vi "FTMS.vi"() -> ()   [LabVIEW 2011]
doc: "Enables and disables RF output of PSG1 & PSG2"
uses:
  Hardware Control/OSC/SubVIs/controls/sampling_rate.ctl
  Hardware Control/OSC/SubVIs/controls/scale.ctl
  global.vi
panel:
  out "frame averages completed:":i32 caption="averages:"
  in  "frame single cycle":bool caption="no averaging"
  in  "reset frame average":bool
  in  "Frame":i32=1 caption="Displayed Frame" min=1 step=1
  out "OSC reading":bool
  in  "meas cluster":T1
  out "waiting":bool
  in  "Pause":bool
  in  "Stop":bool
  out "current step":i32
  out "current frequency":dbl format="%6.2p"
  out "current meas cycle":i32
  out "dt":dbl format="%#_6p"
  out "reset meas cycle timer":bool
  out "first start":bool
  in  "Tab Control":T2(tab)
  in  "EXP chirp end":dbl=1000000000.0 format="%.2p"
  in  "EXP Meas Period (s)":dbl=10.0 min=1.0 format="%.2g"
  in  "Purge Freq.":dbl=2.0 caption="Purge Freq. (Hz)"
  in  "PURGE nozzle":bool
  in  "Refresh meas time":bool
  out "meas cycle time (ms)":u32
  in  "start experiment":bool
  in  "config TRIG":bool
  in  "config OSC":bool
  out "OSC resolution":ext=24999.999999999999998 caption="spectral resolution (Hz)" format="%#_6p"
  out "OSC sample points":i32=200000 caption="points / frame"
  out "TRIG BG cycle":dbl=100.0 caption="BG. cycle" min=0.0 max=999.999999999995 format="%.2p"
  out "TRIG mol delay":dbl=9.999999999999999e-05 caption="Mol. delay" min=0.0 max=999.999999999995 format="%.2p"
  out "TRIG start time":dbl[](array[numeric])=[0.0, 1.1e-06, 6.6e-06, 6.4e-06] caption="delay starts (s)" format="%.3p"
  out "TRIG burst enable":bool=TRUE caption="Burst"
  out "TRIG delay duration":dbl=4.6625e-05 caption="delay cycle (s)" format="%.2p"
  out "TRIG duration":dbl[](array[numeric])=[5.65e-06, 4.9999999999999996e-06, 4e-05, 4.9999999999999996e-06] caption="delay durations (s)" min=0.0 format="%.3p"
  out "TRIG burst period":dbl=4.9999999999999975e-05 caption="burst period (s)" format="%.2p"
  out "TRIG burst count":i32=1 caption="burst count"
  out "horizontal scale":T3=4e-06 items=["400ns/div"=4e-07, "1µs/div"=1e-06, "2µs/div"=2e-06, "4µs/div"=4e-06, "10µs/div"=1e-05, "20µs/div"=2e-05]
  out "sample rate":T4=5000000000.0 items=["20 GHz (50ps/sample)", "10 GHz (100ps/sample)", "5.0 GHz (200ps/sample)", "2.5 GHz (400ps/sample)", "1.25 GHz (0.8ns/sample)", "0.5 GHz (2ns/sample)"]
  in  "EXP Meas Cycles":i32=10 min=1 step=1
  in  "PSG start freq":dbl=0.0003 caption="Start Freq. (Hz)" min=0.00025 max=67.0 step=1e-06 format="%#.12p"
  in  "PSG Amplitude1":dbl caption="PSG1 Ampl (dBm)" min=-135.0 max=30.0 step=0.5 format="%#_8p"
  in  "PSG Amplitude 2":dbl caption="PSG2 Ampl (dBm)" min=-135.0 max=30.0 step=0.5 format="%#_8p"
  in  "PSG freq offset":dbl=0.0003 caption="freq. offset (Hz)" min=0.00025 max=67.0 step=1e-06 format="%#.12p"
  in  "write configs":bool
  in  "load config":bool
  in  "save config":bool
  in  "PSG steps":u32=1 min=1 step=1 format="%.0p"
  in  "PSG step size":dbl=0.0003 caption="step size" min=0.00025 max=67.0 step=1e-06 format="%#.12p"
  out "Meas Time":string="00:00:00"
  out "Experiment Time":string="00:00:00"
  out "meas duration":dbl format="%.1p"
  out "TRIG inhibit off":dbl=9.999999999999999e-05 min=0.0 max=999.999999999995 format="%.1p"
  out "Current Cor Spectra 2":waveform(dbl)(graph) caption="Corrected Frame Time Signal"
  out "Current Background Frame 2":waveform(dbl)(graph) caption="Background Time Signal"
  out "Current Molecular Frame 2":waveform(dbl)(graph) caption="Molecular Time Signal"
  out "Current Molecular Frame":T5(graph) caption="Molecular Frame"
  out "Current Background Frame":T5(graph) caption="Background Frame"
  out "Current Cor Spectra":T5(graph) caption="Corrected Frame"
  out "Average Cor":T5(graph) caption="Average of all corrected time domain signals"
  out "Averaged Background":T5(graph)
  out "Averaged Molecular":T5(graph)
  out "combined spectra":T6(graph)
  out "combined spectra 2":T6(graph)
  in  "Quit":bool
  # "local variables"
  # "General Settings"
  # "PSG Configuration"
  # "TRIG Configuration"
  # "OSC Configuration"
  # "File Storage"
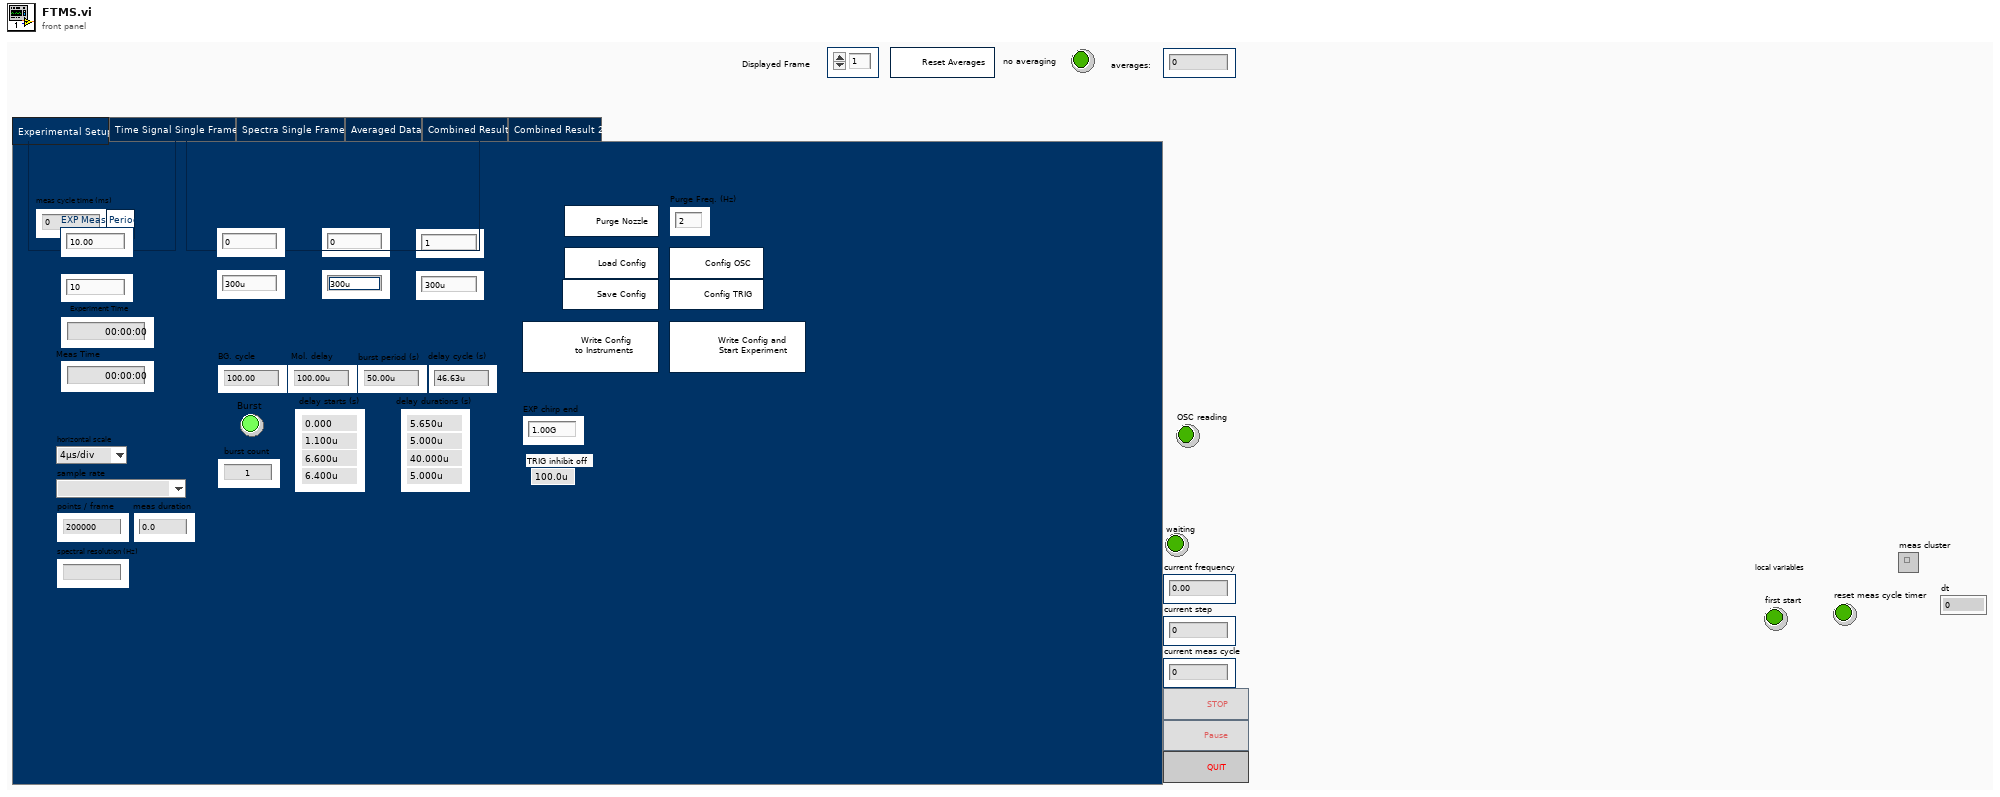
[diagram p1: front panel]
types:
  T1 = cluster{"spectra cluster":cluster{"BG spectrum":cluster{"Numeric Control":dbl, "df":dbl, "magnitude":dbl[]}, "Mol spectrum":cluster{"Numeric Control":dbl, "df":dbl, "magnitude":dbl[]}, "cor spectrum":cluster{"Numeric Control":dbl, "df":dbl, "magnitude":dbl[]}}, "time cluster":cluster{"cor waveform":waveform(dbl), "Mol waveform":waveform(dbl), "BG waveform":waveform(dbl)}}
  T2 = enum32{"Experimental Setup", "Time Signal Single Frames", "Spectra Single Frames", "Averaged Data", "Combined Result", "Combined Result 2"}
  T3 = typedef "scale.ctl" = dbl
  T4 = typedef "sampling_rate.ctl" = ext
  T5 = cluster{"Numeric Control":dbl, "df":dbl, "magnitude":dbl[]}
  T6 = cluster{"Numeric Control":dbl, "df":dbl, "magnitude":dbl[]}[]
  T7 = enum8{"Enabled", "Disabled", "Disabled and Grayed Out"}
  T8 = cluster{"spectra cluster":cluster{"BG spectrum":cluster{"Numeric Control":dbl, "df":dbl, "magnitude":dbl[]}, "Mol spectrum":cluster{"Numeric Control":dbl, "df":dbl, "magnitude":dbl[]}, "cor spectrum":cluster{"Numeric Control":dbl, "df":dbl, "magnitude":dbl[]}}, "time cluster":cluster{"cor waveform":waveform(dbl), "Mol waveform":waveform(dbl), "BG waveform":waveform(dbl)}, "frame cluster":cluster{"wavefrom array":dbl[][], "wavefrom array":dbl[][]}}[]
  T9 = cluster{cluster{"bg waves":waveform(dbl)[], "mol waves":waveform(dbl)[]}, dbl[][][]}
  T10 = cluster{"cor waveform":waveform(dbl), "Mol waveform":waveform(dbl), "BG waveform":waveform(dbl)}
  T11 = cluster{"BG spectrum":cluster{"Numeric Control":dbl, "df":dbl, "magnitude":dbl[]}, "Mol spectrum":cluster{"Numeric Control":dbl, "df":dbl, "magnitude":dbl[]}, "cor spectrum":cluster{"Numeric Control":dbl, "df":dbl, "magnitude":dbl[]}}
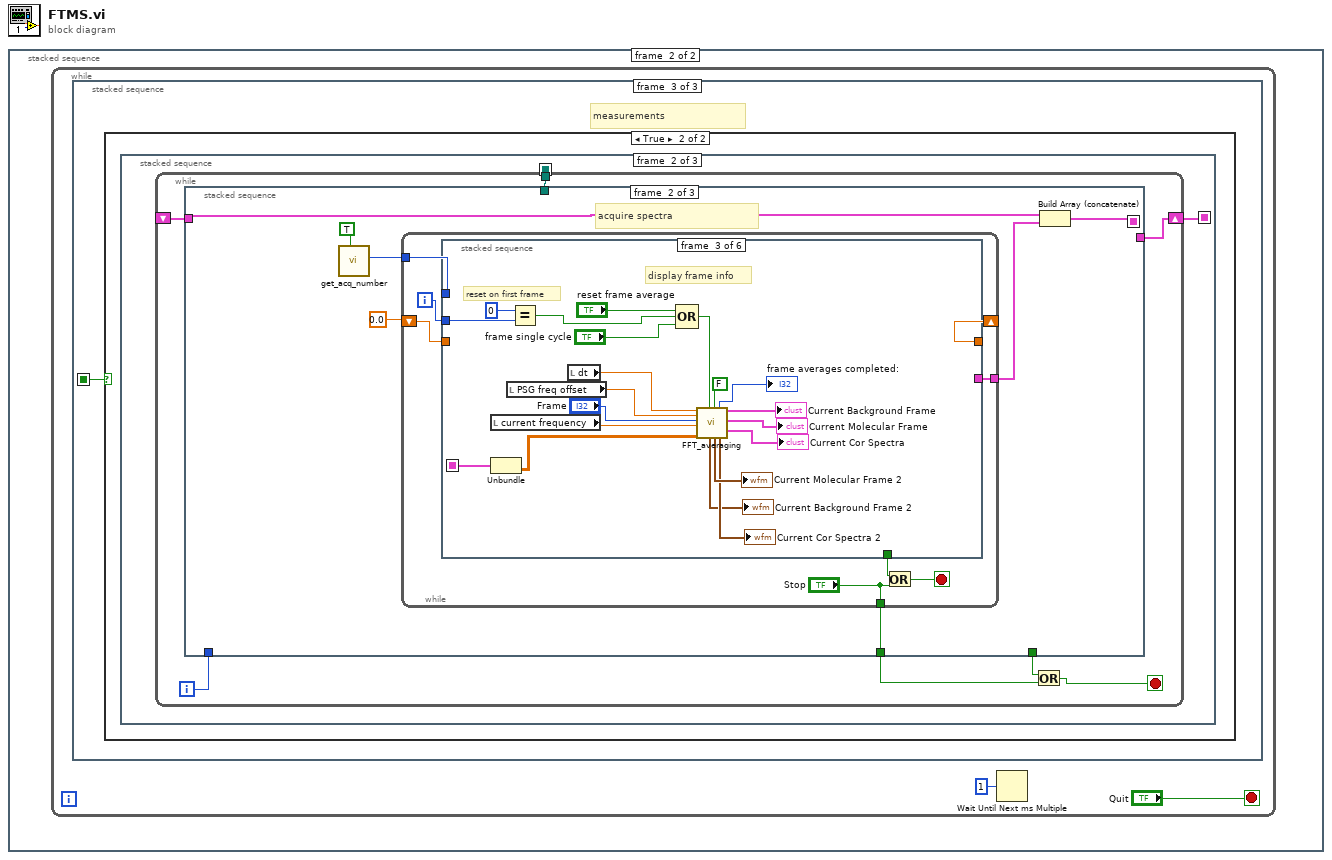
[diagram p0: block diagram]
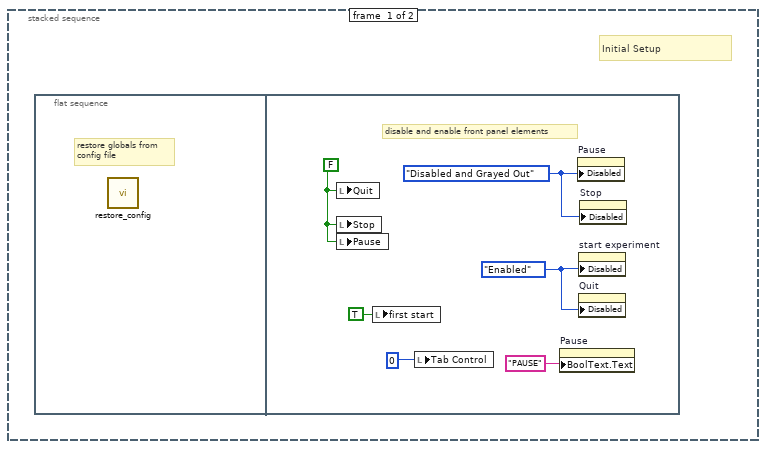
[diagram p2: hidden frame]
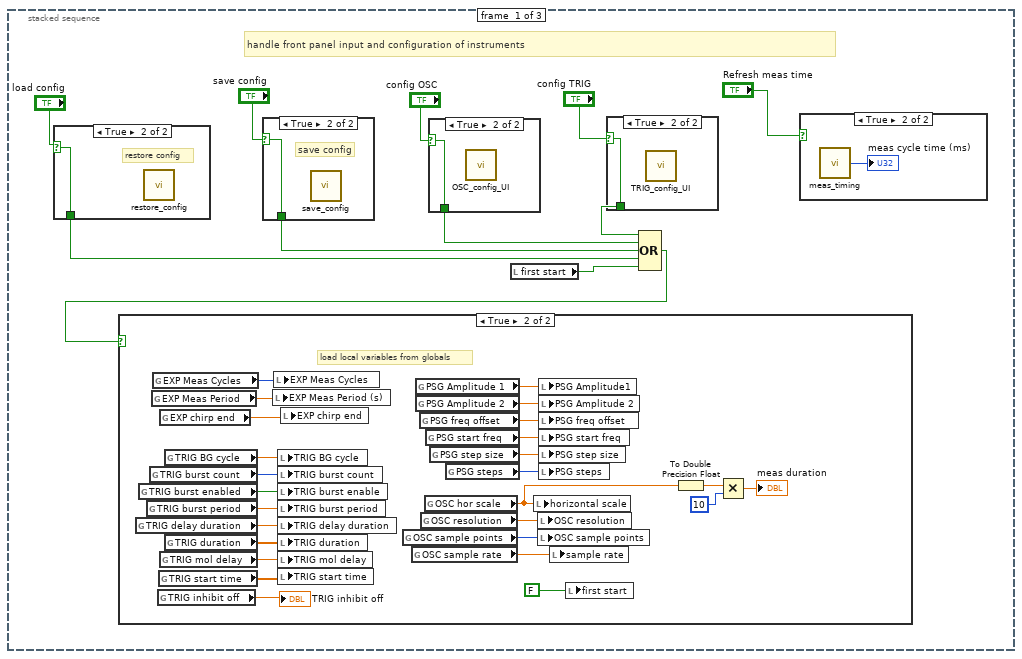
[diagram p3: hidden frame]
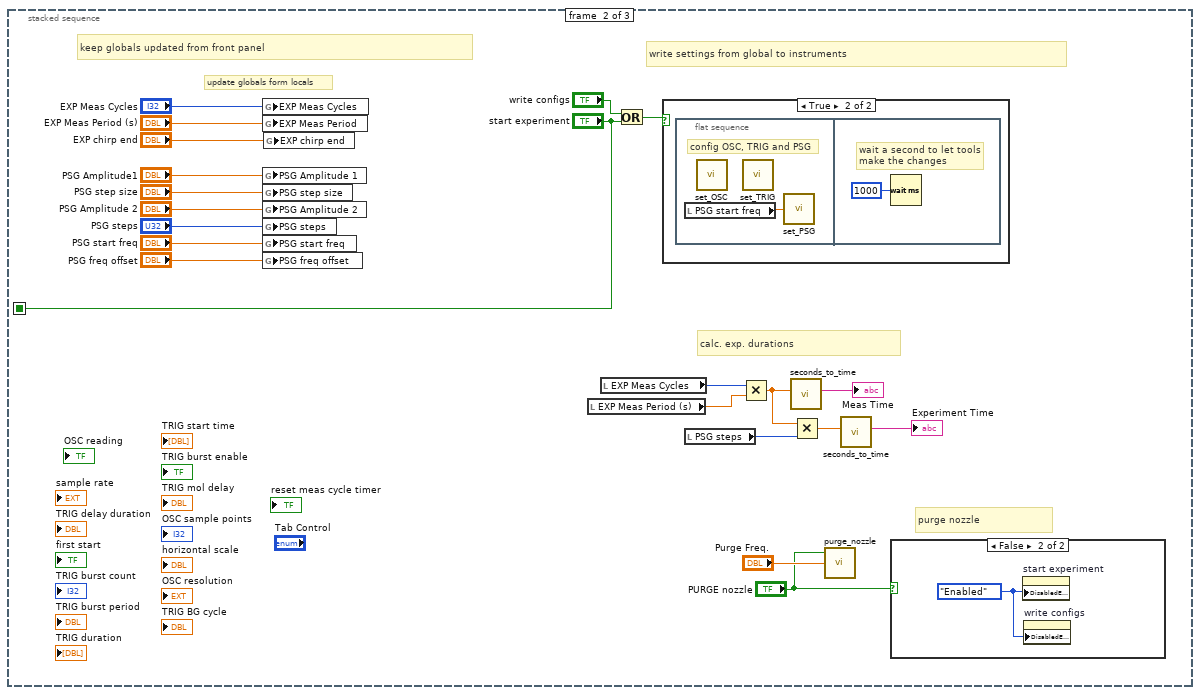
[diagram p10: hidden frame]
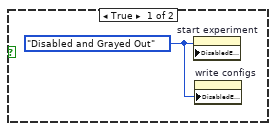
[diagram p11: hidden frame]
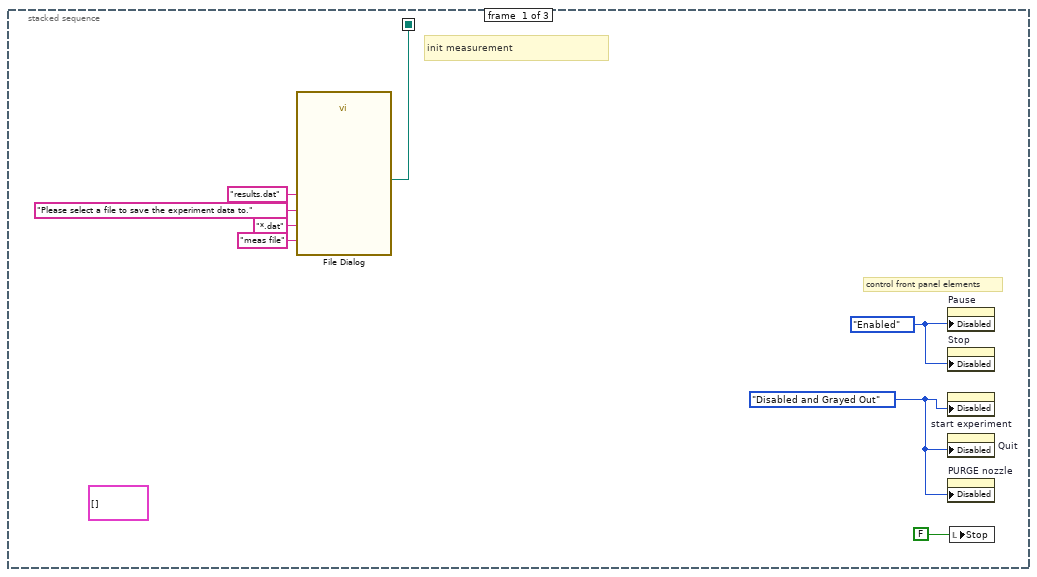
[diagram p14: hidden frame]
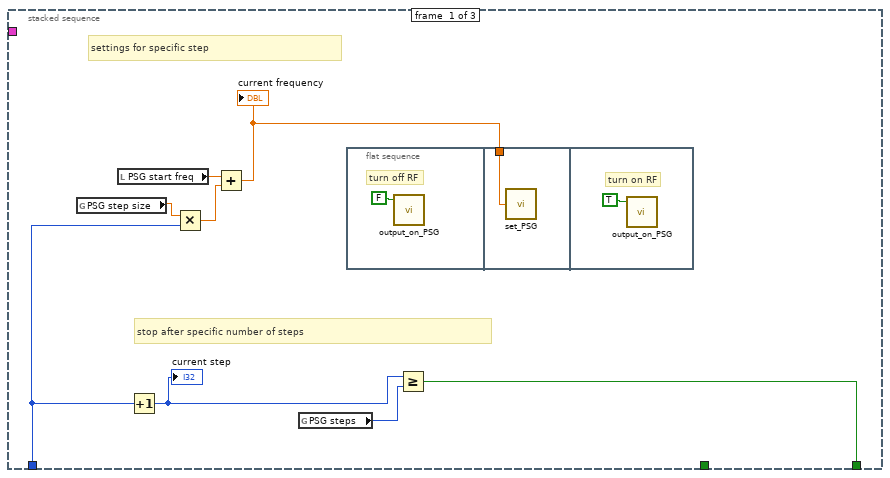
[diagram p15: hidden frame]
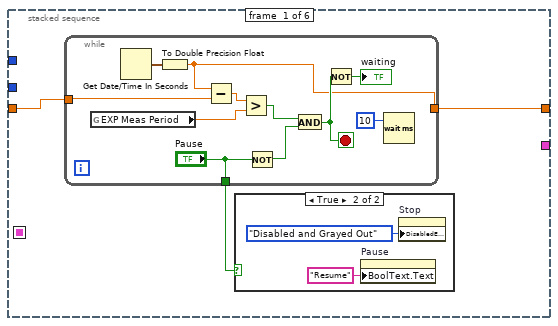
[diagram p16: hidden frame]
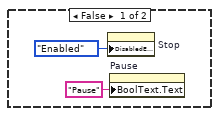
[diagram p17: hidden frame]
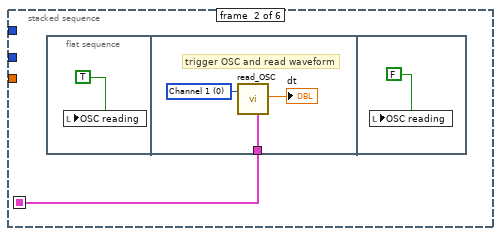
[diagram p18: hidden frame]
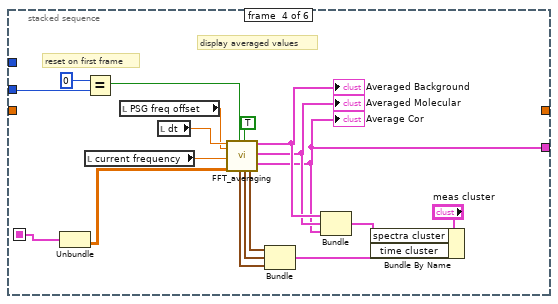
[diagram p19: hidden frame]
diagram:
  n1 = stacked-sequence {
    frame #0 {
      # "Initial Setup"
      n2 = flat-sequence {
        frame #0 {
          # "restore globals from\nconfig file"
          n3 = call "restore_config.vi"() -> ()  [unwired: 5 in]
        }
        frame #1 {
          w5 = T7."Disabled and Grayed Out" ("Disabled")
          w2 = T7."Enabled" ("Disabled")
          w6 = FALSE ("Quit")
          # "disable and enable front panel elements"
          n4 = local write "Quit"(w6) -> ()
          n5 = local write "Stop"(w6) -> ()
          n6 = local write "Pause"(w6) -> ()
          n7 = local write "first start"(TRUE ("first start")) -> ()
          n8 = local write "Tab Control"(0) -> ()
          n9 = property on="Pause" class="Bool (strict)"("BoolText.Text"="PAUSE" ("Boolean Text.Text")) -> ()  [unwired: 2 in, 2 out]
          n10 = property on="Pause" class="Bool (strict)"("Disabled"=w5) -> ()  [unwired: 2 in, 2 out]
          n11 = property on="start experiment" class="Bool"("Disabled"=w2) -> ()  [unwired: 2 in, 2 out]
          n12 = property on="Quit" class="Bool (strict)"("Disabled"=w2) -> ()  [unwired: 2 in, 2 out]
          n13 = property on="Stop" class="Bool (strict)"("Disabled"=w5) -> ()  [unwired: 2 in, 2 out]
        }
      }
    }
    frame #1 {
      n14 = while {
        stop <- "Quit" stop-if-true
        n15 = stacked-sequence {
          seq-local: [_ "start experiment" _] -> [_ _ w80]
          frame #0 {
            # "handle front panel input and configuration of instruments"
            n16 = case shown="True" "load config" {
              selector: "load config" -> [w53 w54]
              tunnel: [w53 w54] -> w11
              frame False {
              }
              frame True {
                # "restore config"
                n17 = call "restore_config.vi"() -> ()  [unwired: 5 in]
              }
            }
            n18 = case shown="True" "save config" {
              selector: "save config" -> [w51 w52]
              tunnel: [w51 w52] -> w13
              frame False {
              }
              frame True {
                # "save config"
                n19 = call "save_config.vi"() -> ()  [unwired: 5 in]
              }
            }
            n20 = case shown="True" "config OSC" {
              selector: "config OSC" -> [w49 w50]
              tunnel: [w49 w50] -> w15
              frame False {
              }
              frame True {
                n21 = call "OSC_config_UI.vi"() -> ()  [unwired: 12 in]
              }
            }
            n22 = local read "first start"() -> (w18:bool)
            n23 = case shown="True" "config TRIG" {
              selector: "config TRIG" -> [w47 w48]
              tunnel: [w47 w48] -> w16
              frame False {
              }
              frame True {
                n24 = call "TRIG_config_UI.vi"() -> ()  [unwired: 12 in]
              }
            }
            n25 = Compound Arithmetic op=OR(w16, w15, w13, w11, w18) -> (w10:bool)
            n26 = case shown="True" w10 {
              frame False {
              }
              frame True {
                # "load local variables from globals"
                n27 = global read "global.vi" "TRIG delay duration"() -> (w32:dbl)
                n28 = global read "global.vi" "TRIG burst enabled"() -> (w34:bool)
                n29 = global read "global.vi" "TRIG burst period"() -> (w33:dbl)
                n30 = global read "global.vi" "TRIG burst count"() -> (w35:i32)
                n31 = global read "global.vi" "EXP Meas Period"() -> (w27:dbl)
                n32 = global read "global.vi" "EXP Meas Cycles"() -> (w46:i32)
                n33 = global read "global.vi" "TRIG inhibit off"() -> (→"TRIG inhibit off":dbl)
                n34 = global read "global.vi" "TRIG start time"() -> (w29:dbl[])
                n35 = global read "global.vi" "EXP chirp end"() -> (w22:dbl)
                n36 = global read "global.vi" "TRIG mol delay"() -> (w30:dbl)
                n37 = global read "global.vi" "TRIG BG cycle"() -> (w36:dbl)
                n38 = global read "global.vi" "TRIG duration"() -> (w31:dbl[])
                n39 = local write "EXP Meas Period (s)"(w27) -> ()
                n40 = local write "EXP Meas Cycles"(w46) -> ()
                n41 = local write "TRIG BG cycle"(w36) -> ()
                n42 = local write "TRIG burst count"(w35) -> ()
                n43 = local write "TRIG burst enable"(w34) -> ()
                n44 = local write "TRIG burst period"(w33) -> ()
                n45 = local write "TRIG delay duration"(w32) -> ()
                n46 = local write "TRIG duration"(w31) -> ()
                n47 = local write "TRIG mol delay"(w30) -> ()
                n48 = local write "TRIG start time"(w29) -> ()
                n49 = local write "EXP chirp end"(w22) -> ()
                n50 = global read "global.vi" "OSC sample points"() -> (w44:i32)
                n51 = global read "global.vi" "OSC sample rate"() -> (w43:T4)
                n52 = global read "global.vi" "PSG Amplitude 1"() -> (w38:dbl)
                n53 = global read "global.vi" "PSG Amplitude 2"() -> (w39:dbl)
                n54 = global read "global.vi" "PSG freq offset"() -> (w40:dbl)
                n55 = global read "global.vi" "OSC resolution"() -> (w45:ext)
                n56 = global read "global.vi" "OSC hor scale"() -> (w23:T3)
                n57 = global read "global.vi" "PSG start freq"() -> (w41:dbl)
                n58 = global read "global.vi" "PSG step size"() -> (w42:dbl)
                n59 = global read "global.vi" "PSG steps"() -> (w37:i32)
                n60 = local write "horizontal scale"(w23) -> ()
                n61 = local write "OSC resolution"(w45) -> ()
                n62 = local write "OSC sample points"(w44) -> ()
                n63 = local write "PSG Amplitude1"(w38) -> ()
                n64 = local write "PSG Amplitude 2"(w39) -> ()
                n65 = local write "PSG freq offset"(w40) -> ()
                n66 = local write "PSG start freq"(w41) -> ()
                n67 = local write "PSG step size"(w42) -> ()
                n68 = local write "PSG steps"(w37) -> ()
                n69 = local write "sample rate"(w43) -> ()
                n70 = local write "first start"(FALSE ("first start")) -> ()
                n71 = To Double Precision Float(number=w23) -> (double precision float=w25:T3)
                n72 = Multiply(x=w25, y=10) -> (x*y=→"meas duration":T3)
              }
            }
            n73 = case shown="True" "Refresh meas time" {
              frame False {
              }
              frame True {
                n74 = call "meas_timing.vi"() -> ("meas cycle time"=→"meas cycle time (ms)":u32)  [unwired: 5 in]
              }
            }
          }
          frame #1 {
            # "calc. exp. durations"
            # "purge nozzle"
            # "write settings from global to instruments"
            # "keep globals updated from front panel"
            # "update globals form locals"
            n75 = global write "global.vi" "EXP Meas Cycles"("EXP Meas Cycles") -> ()
            n76 = global write "global.vi" "EXP Meas Period"("EXP Meas Period (s)") -> ()
            n77 = global write "global.vi" "PSG Amplitude 1"("PSG Amplitude1") -> ()
            n78 = global write "global.vi" "PSG step size"("PSG step size") -> ()
            n79 = global write "global.vi" "PSG Amplitude 2"("PSG Amplitude 2") -> ()
            n80 = global write "global.vi" "PSG steps"("PSG steps") -> ()
            n81 = global write "global.vi" "PSG start freq"("PSG start freq") -> ()
            n82 = global write "global.vi" "PSG freq offset"("PSG freq offset") -> ()
            n83 = global write "global.vi" "EXP chirp end"("EXP chirp end") -> ()
            n84 = local read "EXP Meas Period (s)"() -> (w62:dbl)
            n85 = local read "EXP Meas Cycles"() -> (w63:i32)
            n86 = Or(x="write configs", y="start experiment") -> (x .or. y?=w67:bool)
            n87 = case shown="True" w67 {
              frame False {
              }
              frame True {
                n88 = flat-sequence {
                  frame #0 {
                    # "config OSC, TRIG and PSG"
                    n89 = local read "PSG start freq"() -> (w78:dbl)
                    n90 = call "set_OSC.vi"() -> ()  [unwired: 12 in]
                    n91 = call "set_TRIG.vi"() -> ()  [unwired: 12 in]
                    n92 = call "set_PSG.vi"("PSG1 frequency"=w78) -> ()  [unwired: 5 in]
                  }
                  frame #1 {
                    # "wait a second to let tools \nmake the changes"
                    n93 = Wait (ms)(milliseconds to wait=u32 1000) -> ()  [unwired: 1 out]
                  }
                }
              }
            }
            n94 = local read "PSG steps"() -> (w59:u32)
            n95 = Multiply(x=w63, y=w62) -> (x*y=w60:dbl)
            n96 = call "seconds_to_time.vi"("# Seconds (0)"=w60) -> ("Elapsed Time (00:00:00)"=→"Meas Time":string)  [unwired: 10 in]
            n97 = Multiply(x=w60, y=w59) -> (x*y=w57:dbl)
            n98 = call "purge_nozzle.vi"("purge frequency"="Purge Freq.", "Purge"="PURGE nozzle") -> ()  [unwired: 4 in]
            n99 = call "seconds_to_time.vi"("# Seconds (0)"=w57) -> ("Elapsed Time (00:00:00)"=→"Experiment Time":string)  [unwired: 10 in]
            n100 = case shown="False" "PURGE nozzle" {
              frame True {
                w76 = T7."Disabled and Grayed Out" ("Disabled")
                n101 = property on="start experiment" class="Bool"("DisabledEnum"=w76) -> ()  [unwired: 2 in, 2 out]
                n102 = property on="write configs" class="Bool"("DisabledEnum"=w76) -> ()  [unwired: 2 in, 2 out]
              }
              frame False {
                w77 = T7."Enabled" ("Disabled")
                n103 = property on="start experiment" class="Bool"("DisabledEnum"=w77) -> ()  [unwired: 2 in, 2 out]
                n104 = property on="write configs" class="Bool"("DisabledEnum"=w77) -> ()  [unwired: 2 in, 2 out]
              }
            }
          }
          frame #2 {
            # "measurements"
            n105 = case shown="True" w80 {
              frame False {
              }
              frame True {
                n106 = stacked-sequence {
                  seq-local: [w81 _ _] -> [_ w90 _]
                  seq-local: [_ w89 _] -> [_ _ w197]
                  frame #0 {
                    (unwired) T8 [] ("Array")
                    w88 = T7."Enabled" ("Disabled")
                    w87 = T7."Disabled and Grayed Out" ("Disabled")
                    # "init measurement"
                    # "control front panel elements"
                    n107 = call "File Dialog"("prompt"="Please select a file to save the experiment data to.", "default name"="results.dat", "pattern (all files)"="*.dat", "pattern label"="meas file") -> ("selected path"=w81:path)  [unwired: 8 in, 3 out]
                    n108 = property on="Pause" class="Bool (strict)"("Disabled"=w88) -> ()  [unwired: 2 in, 2 out]
                    n109 = property on="Stop" class="Bool (strict)"("Disabled"=w88) -> ()  [unwired: 2 in, 2 out]
                    n110 = property on="start experiment" class="Bool"("Disabled"=w87) -> ()  [unwired: 2 in, 2 out]
                    n111 = property on="Quit" class="Bool (strict)"("Disabled"=w87) -> ()  [unwired: 2 in, 2 out]
                    n112 = property on="PURGE nozzle" class="Bool (strict)"("Disabled"=w87) -> ()  [unwired: 2 in, 2 out]
                    n113 = local write "Stop"(FALSE ("Stop")) -> ()
                  }
                  frame #1 {
                    n114 = while {
                      tunnel: w90 -> [w93]
                      shift-right: [w91] -> w89
                      shift-left: _ -> [w92]
                      i -> [w97]
                      stop <- w95 stop-if-true
                      n115 = stacked-sequence {
                        seq-local: [_ w110 _] -> [_ _ w191]
                        tunnel: w97 -> [w102 _ _]
                        tunnel: [w101 _ _] -> w96
                        tunnel: [_ w113 _] -> w94
                        tunnel: w93 -> [_ _ w195]
                        tunnel: w92 -> [_ w111 _]
                        tunnel: [_ _ w191] -> w91
                        frame #0 {
                          # "stop after specific number of steps"
                          # "settings for specific step"
                          n116 = global read "global.vi" "PSG step size"() -> (w105:dbl)
                          n117 = local read "PSG start freq"() -> (w104:dbl)
                          n118 = Increment(x=w102) -> (x+1=w99:i32)
                          "current step" <- w99
                          n119 = Multiply(x=w105, y=w102) -> (x*y=w103:dbl)
                          n120 = Add(x=w104, y=w103) -> (x+y=w98:dbl)
                          "current frequency" <- w98
                          n121 = global read "global.vi" "PSG steps"() -> (w100:i32)
                          n122 = flat-sequence {
                            tunnel: w98 -> [w107]
                            frame #0 {
                              # "turn off RF"
                              n123 = call "output_on_PSG.vi"("Enable RF Output (F:Disable)"=FALSE) -> ()  [unwired: 5 in]
                            }
                            frame #1 {
                              n124 = call "set_PSG.vi"("PSG1 frequency"=w107) -> ()  [unwired: 5 in]
                            }
                            frame #2 {
                              # "turn on RF"
                              n125 = call "output_on_PSG.vi"("Enable RF Output (F:Disable)"=TRUE) -> ()  [unwired: 5 in]
                            }
                          }
                          n126 = Greater Or Equal?(x=w99, y=w100) -> (x >= y?=w101:bool)
                        }
                        frame #1 {
                          # "acquire spectra"
                          n127 = call "get_acq_number.vi"("reset acq. number?"=TRUE) -> ("# of meas cycles"=w114:i32)  [unwired: 7 in, 3 out]
                          n128 = while {
                            tunnel: w114 -> [w122]
                            shift-right: [w120] -> _
                            shift-left: 0.0 -> [w119]
                            tunnel: ["Stop"] -> w113
                            tunnel: [w116] -> w112
                            i -> [w123]
                            stop <- w118 stop-if-true
                            n129 = stacked-sequence {
                              seq-local: [_ w142 _ _ _ _] -> [_ _ w152 w169 _ _]
                              tunnel: w123 -> [_ _ w162 w183 _ _]
                              tunnel: w122 -> [_ _ _ _ _ w189]
                              tunnel: [_ _ _ _ _ w188] -> w121
                              tunnel: [w126 _ _ _ _ _] -> w120
                              tunnel: w119 -> [w125 _ _ _ _ _]
                              tunnel: [_ _ _ w171 _ _] -> w116
                              frame #0 {
                                n130 = while {
                                tunnel: [w134] -> w126
                                tunnel: w125 -> [w140]
                                tunnel: ["Pause"] -> w124
                                stop <- w136 stop-if-true
                                n131 = global read "global.vi" "EXP Meas Period"() -> (w138:dbl)
                                n132 = Get Date/Time In Seconds() -> (seconds since 1Jan1904=w141:timestamp)
                                n133 = To Double Precision Float(number=w141) -> (double precision float=w134:dbl)
                                n134 = Subtract(x=w134, y=w140) -> (x-y=w139:dbl)
                                n135 = Greater?(x=w139, y=w138) -> (0:w133:bool)
                                n136 = Not(x="Pause") -> (.not. x?=w132:bool)
                                n137 = And(x=w133, y=w132) -> (x .and. y?=w136:bool)
                                n138 = Not(x=w136) -> (.not. x?=→"waiting":bool)
                                n139 = Wait (ms)(milliseconds to wait=u32 10) -> ()  [unwired: 1 out]
                                }
                                n140 = case shown="True" w124 {
                                frame False {
                                n141 = property on="Stop" class="Bool (strict)"("DisabledEnum"=T7."Enabled" ("Disabled")) -> ()  [unwired: 2 in, 2 out]
                                n142 = property on="Pause" class="Bool (strict)"("BoolText.Text"="Pause" ("Caption.Text")) -> ()  [unwired: 2 in, 2 out]
                                }
                                frame True {
                                n143 = property on="Pause" class="Bool (strict)"("BoolText.Text"="Resume" ("Caption.Text")) -> ()  [unwired: 2 in, 2 out]
                                n144 = property on="Stop" class="Bool (strict)"("DisabledEnum"=T7."Disabled and Grayed Out" ("Disabled")) -> ()  [unwired: 2 in, 2 out]
                                }
                                }
                              }
                              frame #1 {
                                n145 = flat-sequence {
                                tunnel: [w146] -> w142
                                frame #0 {
                                n146 = local write "OSC reading"(TRUE) -> ()
                                }
                                frame #1 {
                                w145 = u16 0 items=["Channel 1", "Channel 2", "Channel 3", "Channel 4", "Math 1", "Math 2", "Math 3", "Math 4", "Reference 1", "Reference 2", "Reference 3", "Reference 4"] ("Channel (0: Channel 1)")
                                # "trigger OSC and read waveform"
                                n147 = call "read_OSC.vi"("Channel (0: Channel 1)"=w145) -> ("output cluster"=w146:T9, "dt"=→"dt":dbl)  [unwired: 7 in, 2 out]
                                }
                                frame #2 {
                                n148 = local write "OSC reading"(FALSE) -> ()
                                }
                                }
                              }
                              frame #2 {
                                # "reset on first frame"
                                # "display frame info"
                                n149 = local read "current frequency"() -> (w166:dbl)
                                n150 = Unbundle(w152) -> (w151:dbl[][][])  [unwired: 1 out]
                                n151 = local read "PSG freq offset"() -> (w153:dbl)
                                n152 = Equal?(x=0, y=w162) -> (x = y?=w159:bool)
                                n153 = local read "dt"() -> (w167:dbl)
                                n154 = Compound Arithmetic op=OR("reset frame average", w159, "frame single cycle") -> (w157:bool)
                                n155 = call "FFT_averaging.vi"("dt"=w167, "freq. offset"=w153, "frame"="Frame", "current frequency"=w166, "3d waveform array"=w151, "reset frame average"=w157, "all frames?"=FALSE) -> ("BG waveform"=→"Current Background Frame 2":waveform(dbl), "Mol waveform"=→"Current Molecular Frame 2":waveform(dbl), "averages compl"=→"frame averages completed:":i32, "cor waveform"=→"Current Cor Spectra 2":waveform(dbl), "BG spectrum"=→"Current Background Frame":T5, "Mol spectrum"=→"Current Molecular Frame":T5, "cor spectrum"=→"Current Cor Spectra":T5)  [unwired: 6 in]
                              }
                              frame #3 {
                                # "reset on first frame"
                                # "display averaged values"
                                n156 = Unbundle(w169) -> (w168:dbl[][][])  [unwired: 1 out]
                                n157 = Equal?(x=0, y=w183) -> (x = y?=w180:bool)
                                n158 = local read "current frequency"() -> (w181:dbl)
                                n159 = local read "PSG freq offset"() -> (w170:dbl)
                                n160 = local read "dt"() -> (w182:dbl)
                                n161 = call "FFT_averaging.vi"("dt"=w182, "freq. offset"=w170, "current frequency"=w181, "3d waveform array"=w168, "reset frame average"=w180, "all frames?"=TRUE) -> ("BG waveform"=w175:waveform(dbl), "Mol waveform"=w176:waveform(dbl), "cor waveform"=w177:waveform(dbl), "BG spectrum"=w179:T5, "Mol spectrum"=w178:T5, "cor spectrum"=w171:T5)  [unwired: 7 in, 1 out]
                                "Average Cor" <- w171
                                "Averaged Background" <- w179
                                "Averaged Molecular" <- w178
                                n162 = Bundle("cor waveform"=w177, "Mol waveform"=w176, "BG waveform"=w175) -> (w172:T10)  [unwired: 1 in]
                                n163 = Bundle ("bundle time domain data")("BG spectrum"=w179, "Mol spectrum"=w178, "cor spectrum"=w171) -> (w173:T11)  [unwired: 1 in]
                                n164 = Bundle By Name(cluster="meas cluster", "spectra cluster"=w173, "time cluster"=w172) -> ()  [unwired: 1 out]
                              }
                              frame #4 {
                                # "save frames seperately"
                              }
                              frame #5 {
                                # "stop after N meas cycles or when \nstop is pressed"
                                n165 = global read "global.vi" "EXP Meas Cycles"() -> (w186:i32)
                                n166 = call "get_acq_number.vi"() -> ("# of meas cycles"=w190:i32)  [unwired: 8 in, 3 out]
                                n167 = Subtract(x=w190, y=w189) -> (x-y=w187:i32)
                                "current meas cycle" <- w187
                                n168 = Greater Or Equal?(x=w187, y=w186) -> (x >= y?=w188:bool)
                              }
                            }
                            n169 = Or(x=w121, y="Stop") -> (x .or. y?=w118:bool)
                          }
                          n170 = Build Array (concatenate)(w111, w112) -> (w110:T6)
                        }
                        frame #2 {
                          # "save between steps as backup, overwrite old files"
                          n171 = Strip Path(path=w195) -> (stripped path=w194:path)  [unwired: 1 out]
                          n172 = Build Path(base path=w194, name or relative path="temp") -> (appended path=w192:path)
                          n173 = Build Path(base path=w192, name or relative path="temp_corrected_spectrum.dat") -> ()  [unwired: 1 out]
                          "combined spectra" <- w191
                        }
                      }
                      n174 = Or(x=w96, y=w94) -> (x .or. y?=w95:bool)
                    }
                  }
                  frame #2 {
                    w201 = T7."Disabled and Grayed Out" ("Disabled")
                    w200 = T7."Enabled" ("Disabled")
                    # "turn off RF"
                    n175 = local write "Stop"(FALSE ("Stop")) -> ()
                    n176 = call "output_on_PSG.vi"("Enable RF Output (F:Disable)"=FALSE) -> ()  [unwired: 5 in]
                    n177 = property on="Pause" class="Bool (strict)"("Disabled"=w201) -> ()  [unwired: 2 in, 2 out]
                    n178 = property on="Stop" class="Bool (strict)"("Disabled"=w201) -> ()  [unwired: 2 in, 2 out]
                    n179 = property on="start experiment" class="Bool"("Disabled"=w200) -> ()  [unwired: 2 in, 2 out]
                    n180 = property on="Quit" class="Bool (strict)"("Disabled"=w200) -> ()  [unwired: 2 in, 2 out]
                    n181 = property on="PURGE nozzle" class="Bool (strict)"("Disabled"=w200) -> ()  [unwired: 2 in, 2 out]
                    "combined spectra 2" <- w197
                  }
                }
              }
            }
          }
        }
        n182 = Wait Until Next ms Multiple(millisecond multiple=u32 1) -> ()  [unwired: 1 out]
      }
    }
  }
